vi "OE1022D_Configure Trigger.vi"(2 "VISA resource name":refnum<visa-resource-name>, 3 "Trigger Source (0: Internal)":u16(ring) items=["Internal", "External"]) -> ()   [LabVIEW 2024]
doc: "Configures the reference source and the internal oscillator."
uses:
  Stanford Research 830/Stanford Research 830.lvlib
panel:
  out "VISA resource name out":refnum<visa-resource-name>
  out "error out":errorcluster
  in  "error in (no error)":errorcluster
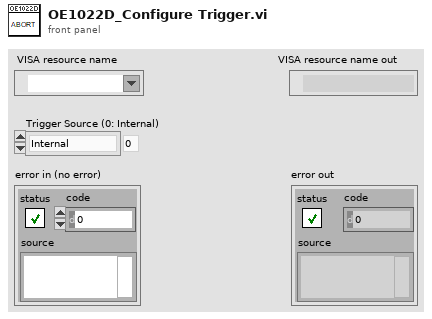
[diagram p1: front panel]
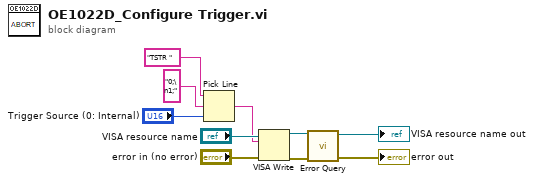
[diagram p0: block diagram]
diagram:
  n1 = Pick Line(string ("")="TSTR ", multi-line string="0;\n1;", line index="Trigger Source (0: Internal)") -> (output string=w5:string)
  n2 = VISA Write(VISA resource name="VISA resource name", write buffer=w5, error in (no error)="error in (no error)") -> (VISA resource name out=w4:refnum<visa-resource-name>, error out=w3:errorcluster)  [unwired: 1 out]
  n3 = call "Error Query.vi"("error in (no error)"=w3, "VISA resource name"=w4) -> ("error out"=→"error out":errorcluster, "VISA resource name out"=→"VISA resource name out":refnum<visa-resource-name>)  [unwired: 7 in, 1 out]
